vi "Initialization.vi"(4 "TestPanel":refnum<vi>, 6 "PIDAdj":refnum<vi>, 7 "TorqueUnit":string, 8 "error in (no error)":errorcluster, 9 "ComponentsRefs":refnum<vi>[](array[refnum]), 10 "TestType":enum16{"Normal", "Stall"}(ring), 11 "TestMultiPtProc in":refnum<class "TestMultiPtProc.lvclass">) -> (0 "error out":errorcluster, 3 "TestMultiPtProc out":refnum<class "TestMultiPtProc.lvclass">)   [LabVIEW 2024, in "TestMultiPtActor.lvlib" / "TestMultiPtProc.lvclass"]
uses:
  TestMultiPtProc.lvclass
  TestMultiPtProc.lvclass/TestMultiPtProc.ctl
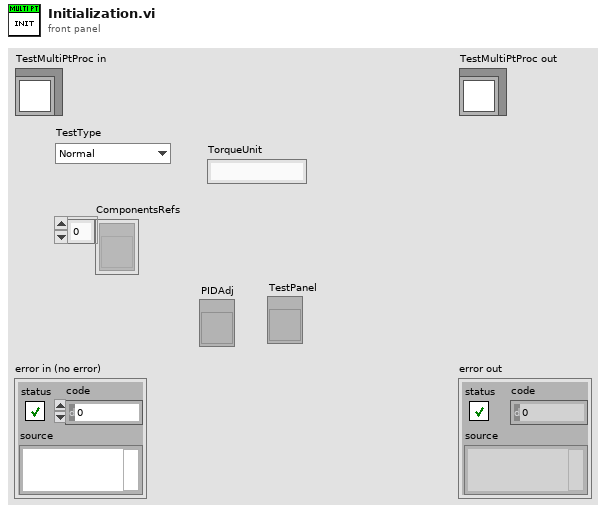
[diagram p1: front panel]
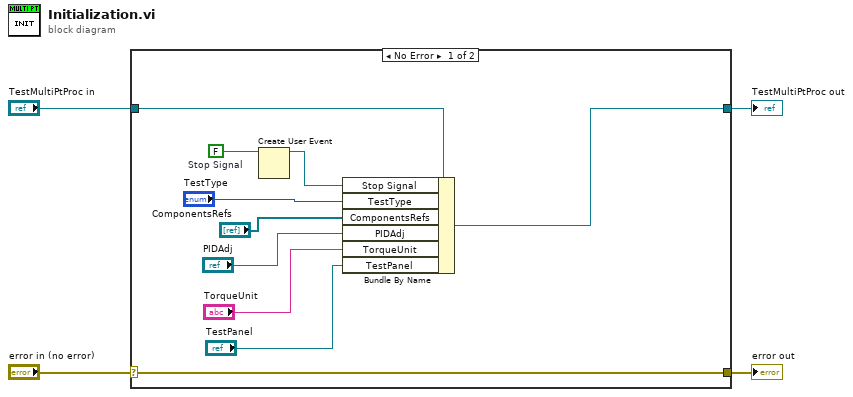
[diagram p0: block diagram]
diagram:
  n1 = case shown="No Error" "error in (no error)" {
    selector: "error in (no error)" -> [w14 w16]
    tunnel: [w14 w16] -> w3
    tunnel: [w7 w15] -> w1
    tunnel: "TestMultiPtProc in" -> [w8 w15]
    frame No Error {
      w13 = FALSE  # Stop Signal
      n2 = Create User Event(user event datatype=w13) -> (user event=w12:refnum<user-event>)  [unwired: 1 in, 1 out]
      n3 = Bundle By Name(cluster=w8, "Stop Signal"=w12, "TestType"="TestType", "ComponentsRefs"="ComponentsRefs", "PIDAdj"="PIDAdj", "TorqueUnit"="TorqueUnit", "TestPanel"="TestPanel") -> (w7:refnum<class "TestMultiPtProc.lvclass">)
    }
    frame Error {
    }
  }
  "error out" <- w3
  "TestMultiPtProc out" <- w1
